vi "Scan Nodes.vi"() -> (0 "error out":errorcluster)   [LabVIEW 2021]
uses:
  Zenoh.lvclass/Zenoh.ctl
  Wrappers/Scan Nodes Wrapper.vi
  SubVIs/Get Zenoh Path.vi
  Zenoh.lvclass
panel:
  out "Nodes":string[](array[string])
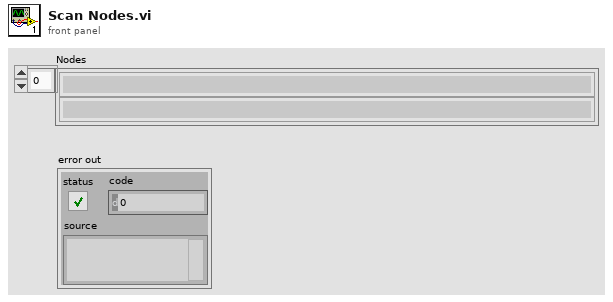
[diagram p1: front panel]
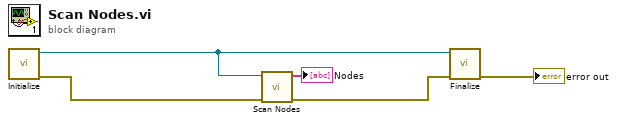
[diagram p0: block diagram]
diagram:
  n1 = call "Initialize.vi"() -> ("error out"=w3:errorcluster, "Zenoh out"=w4:refnum<class "Zenoh.lvclass">)  [unwired: 10 in]
  n2 = call "Scan Nodes.vi"("error in (no error)"=w3, "Zenoh in"=w4) -> ("error out"=w2:errorcluster, "Nodes"=→"Nodes":string[])  [unwired: 8 in]
  n3 = call "Finalize.vi"("error in (no error)"=w2, "Zenoh in"=w4) -> ("error out"=→"error out":errorcluster)  [unwired: 8 in, 1 out]
